vi "cmamo.vi"() -> ()   [LabVIEW 2015]
panel:
  in  "stop":bool
  in  "Consumo Litros/Segundo":dbl(slide) scale=0.0..1.0
  out "Grafico nivel de agua sobre tiempo":dbl(graph)
  out "Tank":dbl(slide) scale=0.0..200.0
  out "NIVEL":dbl
  out "Multi-Segment Pipe":bool(c317)
  in  "Nivel Bajo":dbl
  in  "Nivel Alto":dbl
  out "Bomba":bool
  out "Boolean 2":bool
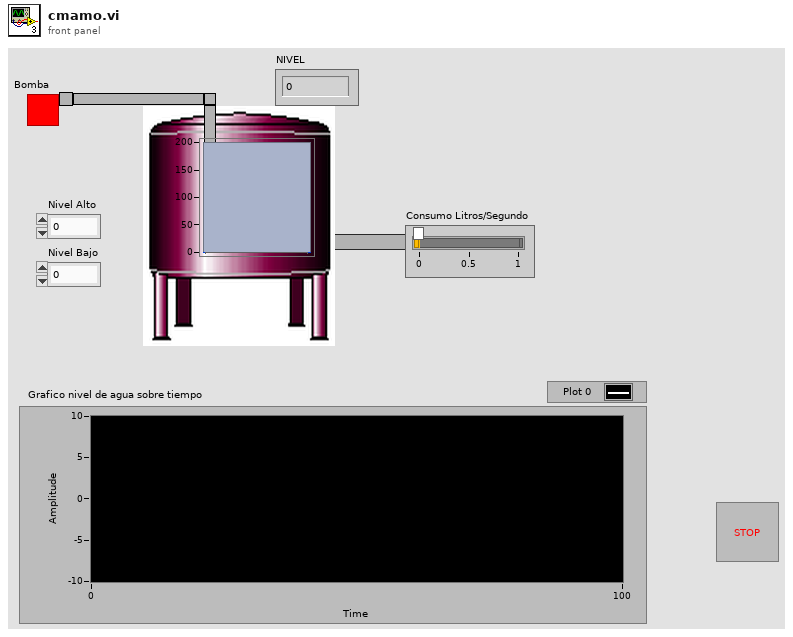
[diagram p1: front panel]
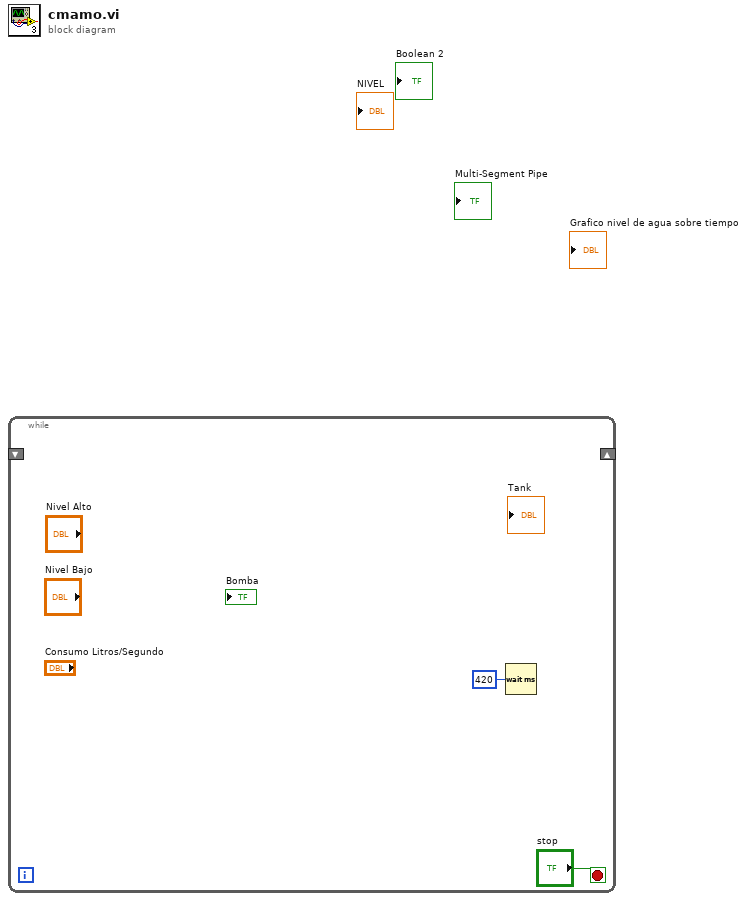
[diagram p0: block diagram]
diagram:
  n1 = while {
    shift-right: _ -> [_]
    shift-left: _ -> [_]
    stop <- "stop" stop-if-true
    n2 = Wait (ms)(milliseconds to wait=u32 420) -> ()  [unwired: 1 out]
  }
